vi "Greater_Array.vi"() -> ()   [LabVIEW 2024]
panel:
  out "Output Array":dbl[][](array[numeric])
  out "Greater Number":dbl[](array[numeric])
  out "Random Number 2":dbl[](array[numeric])
  out "Random Number 1":dbl[](array[numeric])
  in  "Numeric":i32
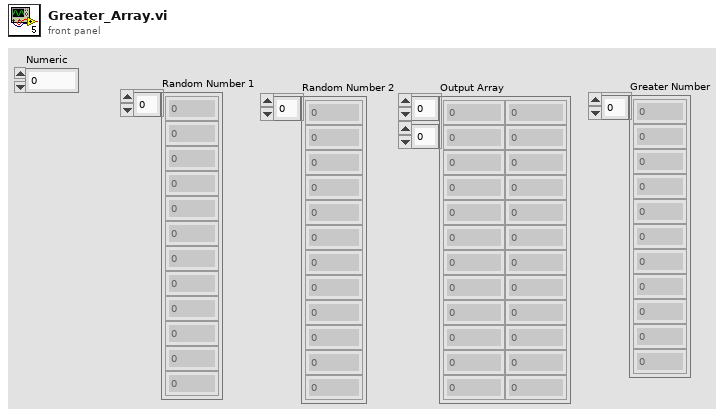
[diagram p1: front panel]
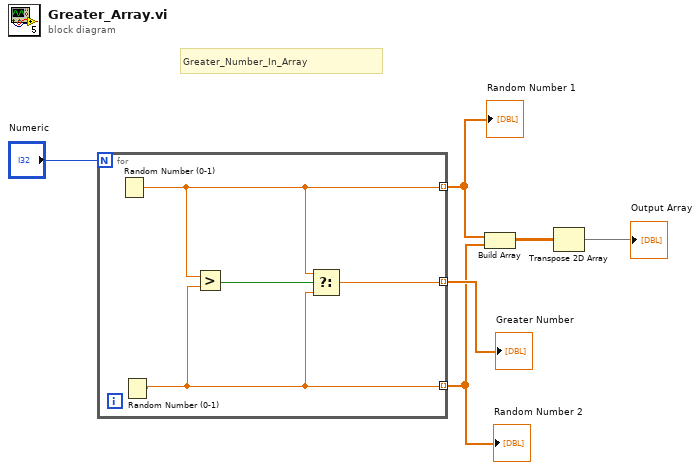
[diagram p0: block diagram]
diagram:
  # "Greater_Number_In_Array"
  n1 = for {
    N: "Numeric" -> [_]
    tunnel: [w8] -> w3 mode=indexing
    tunnel: [w7] -> w4 mode=indexing
    tunnel: [w9] -> w5 mode=indexing
    n2 = Random Number (0-1)() -> (number: 0 to 1=w8:dbl)
    n3 = Random Number (0-1)() -> (number: 0 to 1=w7:dbl)
    n4 = Greater?(x=w8, y=w7) -> (0:w10:bool)
    n5 = Select(t=w8, s=w10, f=w7) -> (s? t:f=w9:dbl)
  }
  "Random Number 1" <- w3
  "Random Number 2" <- w4
  "Greater Number" <- w5
  n6 = Build Array(w3, w4) -> (w2:dbl[][])
  n7 = Transpose 2D Array(2D array=w2) -> (transposed array=→"Output Array":dbl[][])
